vi "HXG2-Error_Module.vi"(6 "user event out":refnum<user-event>, 7 "Command (Handle Errors)":T1=enum."Handle", 8 "error in (no error)":errorcluster, 9 "DAQ Q":refnum<queue>, 10 "Main Q":refnum<queue>, 11 "notifier":refnum<notifier>) -> (0 "error out":errorcluster, 2 "status":bool)   [LabVIEW 2012]
doc: "If an error occurs, this module will gracefully shut down the TLC application by stopping the producer, consumer, and display loops."
uses:
  HXG2-Error_Module.ctl
  Controls/UI/HXG2_MainStateCtrl.ctl
  Controls/HXG2_DAQLOOPctrl.ctl
panel:
  # "Output"
  # "Input"
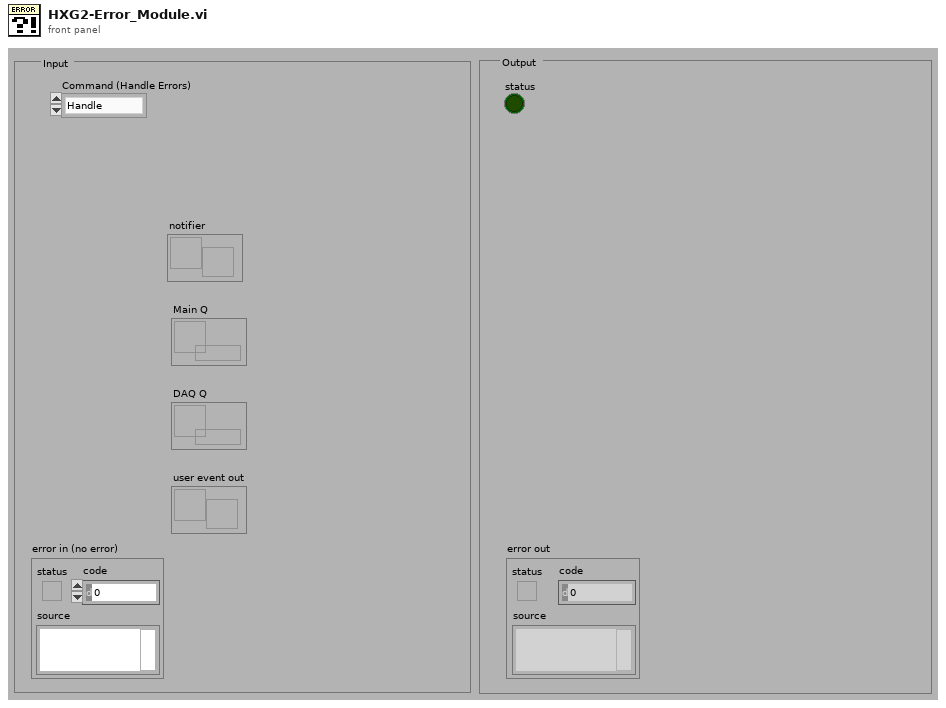
[diagram p1: front panel]
types:
  T1 = typedef "HXG2-Error_Module.ctl" = enum16{"Initialize", "Handle", "Report"}
  T2 = typedef "HXG2_DAQLOOPctrl.ctl" = enum16{"Initialize", "DAQ", "Stop"}
  T3 = typedef "HXG2_MainStateCtrl.ctl" = enum16{"Initialize", "Initialize UI", "DAQ", "Process", "Control", "Write", "Save", "Print", "Graph", "Sequencer", "ERROR", "Exit"}
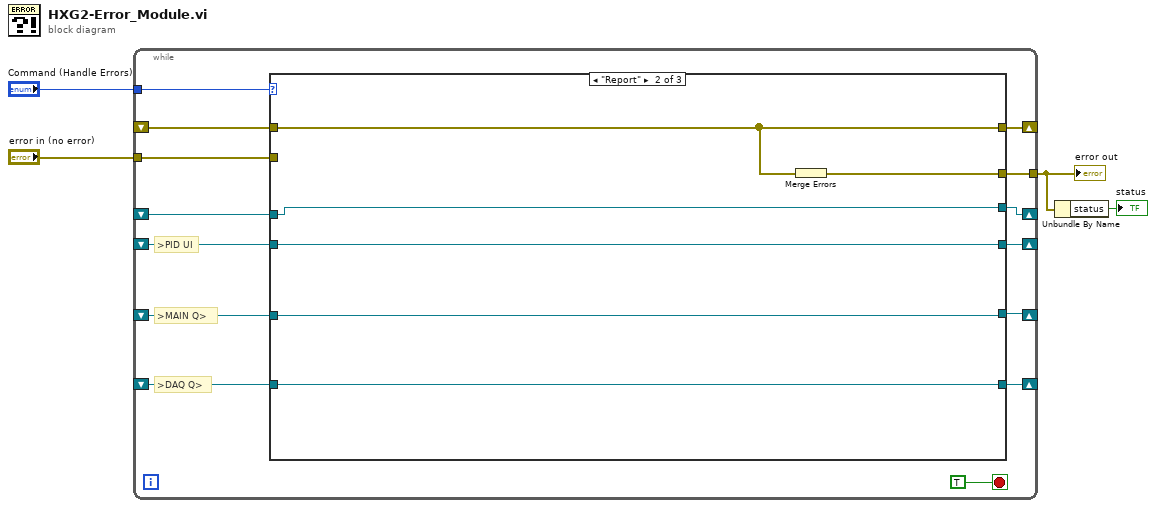
[diagram p0: block diagram]
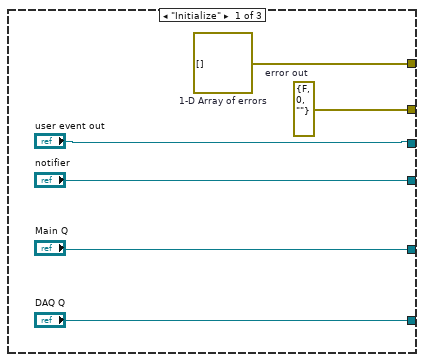
[diagram p2: hidden frame]
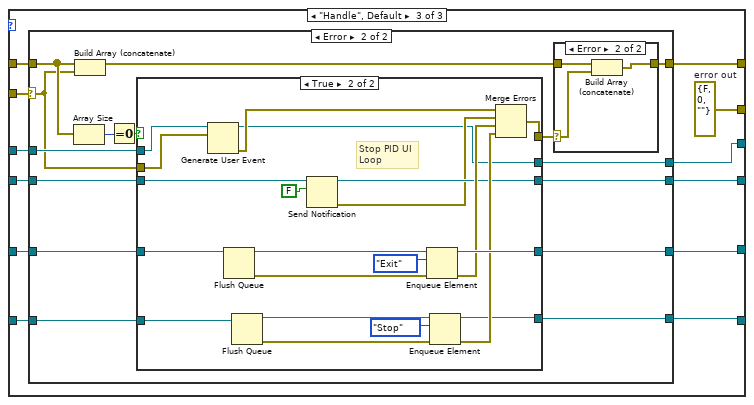
[diagram p3: hidden frame]
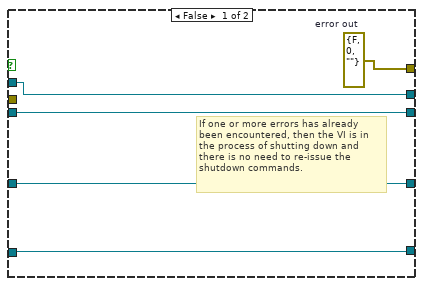
[diagram p6: hidden frame]
diagram:
  n1 = while {
    shift-right: [w14] -> _
    shift-left: _ -> [w16]
    tunnel: "error in (no error)" -> [w17]
    tunnel: "Command (Handle Errors)" -> [w15]
    tunnel: [w13] -> w2
    shift-right: [w12] -> _
    shift-left: _ -> [w9]
    shift-right: [w11] -> _
    shift-left: _ -> [w8]
    shift-right: [w10] -> _
    shift-left: _ -> [w7]
    shift-right: [w5] -> _
    shift-left: _ -> [w6]
    stop <- TRUE stop-if-true
    # ">DAQ Q>"
    # ">MAIN Q>"
    # ">PID UI"
    n2 = case shown="\"Report\"" w15 {
      tunnel: w17 -> [_ _ w42]
      tunnel: [w24 w29 w40] -> w14
      tunnel: w16 -> [_ w29 w41]
      tunnel: [w23 w30 w39] -> w13
      tunnel: ["notifier" w28 w33] -> w12
      tunnel: ["Main Q" w27 w34] -> w11
      tunnel: ["DAQ Q" w26 w35] -> w10
      tunnel: w9 -> [_ w28 w38]
      tunnel: w8 -> [_ w27 w37]
      tunnel: w7 -> [_ w26 w36]
      tunnel: w6 -> [_ w25 w32]
      tunnel: ["user event out" w25 w31] -> w5
      frame "Initialize" {
        w23 = errorcluster {"status"=FALSE, "code"=0, "source"=""}  # error out
        w24 = errorcluster[] []  # 1-D Array of errors
      }
      frame "Report" {
        n3 = Merge Errors(w29) -> (w30:errorcluster)
      }
      frame "Handle", Default {
        w39 = errorcluster {"status"=FALSE, "code"=0, "source"=""}  # error out
        n4 = case shown="Error" w42 {
          selector: w42 -> [_ w48]
          tunnel: [w47 w58] -> w40
          tunnel: w41 -> [w47 w62]
          tunnel: w38 -> [w46 w56]
          tunnel: w37 -> [w45 w55]
          tunnel: w36 -> [w44 w54]
          tunnel: [w44 w53] -> w35
          tunnel: [w45 w52] -> w34
          tunnel: [w46 w51] -> w33
          tunnel: w32 -> [w43 w50]
          tunnel: [w43 w49] -> w31
          frame No Error {
          }
          frame Error {
            n5 = Array Size(array=w62) -> (size(s)=w60:i32)
            n6 = Build Array (concatenate)(w62, w48) -> (w59:errorcluster[])
            n7 = Equal To 0?(x=w60) -> (x = 0?=w61:bool)
            n8 = case shown="True" w61 {
              tunnel: [w71 w88] -> w57
              tunnel: w56 -> [w70 w81]
              tunnel: w55 -> [w69 w92]
              tunnel: w54 -> [w68 w86]
              tunnel: [w68 w82] -> w53
              tunnel: [w69 w89] -> w52
              tunnel: [w70 w80] -> w51
              tunnel: w50 -> [w67 w75]
              tunnel: [w67 w73] -> w49
              tunnel: w48 -> [_ w72]
              frame False {
                w71 = errorcluster {"status"=FALSE, "code"=0, "source"=""}  # error out
                # "If one or more errors has already \nbeen encountered, then the VI is in \nthe process of shutting down and \nthere is no need to re-issue the \nshutdown commands."
              }
              frame True {
                # "Stop PID UI\nLoop"
                n9 = Generate User Event(user event=w75, event data cluster=w72) -> (user event out=w73:refnum<user-event>, error out=w74:errorcluster)  [unwired: 1 in]
                n10 = Flush Queue(queue=w92) -> (queue out=w91:refnum<queue>, error out=w90:errorcluster)  [unwired: 1 in, 1 out]
                n11 = Flush Queue(queue=w86) -> (queue out=w85:refnum<queue>, error out=w84:errorcluster)  [unwired: 1 in, 1 out]
                n12 = Send Notification(notification=FALSE, notifier=w81) -> (notifier out=w80:refnum<notifier>, error out=w79:errorcluster)  [unwired: 1 in]
                n13 = Enqueue Element(queue=w91, element=HXG2_MainStateCtrl."Exit", error in (no error)=w90) -> (queue out=w89:refnum<queue>, error out=w87:errorcluster)  [unwired: 1 in, 1 out]
                n14 = Enqueue Element(queue=w85, element=HXG2_DAQLOOPctrl."Stop", error in (no error)=w84) -> (queue out=w82:refnum<queue>, error out=w83:errorcluster)  [unwired: 1 in, 1 out]
                n15 = Merge Errors(w74, w79, w87, w83) -> (w88:errorcluster)
              }
            }
            n16 = case shown="Error" w57 {
              selector: w57 -> [_ w64]
              tunnel: w59 -> [w63 w66]
              tunnel: [w63 w65] -> w58
              frame No Error {
              }
              frame Error {
                n17 = Build Array (concatenate)(w66, w64) -> (w65:errorcluster[])
              }
            }
          }
        }
      }
    }
  }
  "error out" <- w2
  n18 = Unbundle By Name(w2) -> ("status"=→"status":bool)
